vi "Handle Value Change.vi"(5 "VolatusAPI":refnum<class "VolatusAPI.lvclass">, 7 "CtlRef":refnum<vi>, 8 "error in (no error)":errorcluster, 9 "NewVal":variant, 10 "OldVal":variant, 11 "BooleanControl in":refnum<class "BooleanControl.lvclass">) -> (0 "error out":errorcluster, 3 "BooleanControl out":refnum<class "BooleanControl.lvclass">)   [LabVIEW 2020, in "VolatusGUIElements.lvlib" / "BooleanControl.lvclass"]
uses:
  BooleanControl.lvclass
  BooleanControl.lvclass/BooleanControl.ctl
  messages/CmdDigital/Data.ctl
  messages/CmdDigital/CmdDigital.lvlib
  messages/CmdDigital/Class/Msg.lvclass
  Volatus/VolatusAPI/VolatusAPI.lvclass
  VolatusGUI/GUI Element/GUI Element.lvclass
  C:/dev/lv20CE/relink/lv-volatus/messages/CmdDigital/Class/Msg.lvclass
  C:/dev/lv20CE/relink/lv-protoc/LV-Proto/Message/Message.lvclass
  C:/dev/lv20CE/relink/lv-volatus/VolatusGUI/GUI Element/GUI Element.lvclass
  C:/dev/lv20CE/relink/lv-volatus/VolatusGUIElements/BooleanControl/BooleanControl.lvclass
  C:/dev/lv20CE/relink/lv-volatus/VolatusGUI/OnValueChangeHandler/OnValueChangeHandler.lvclass
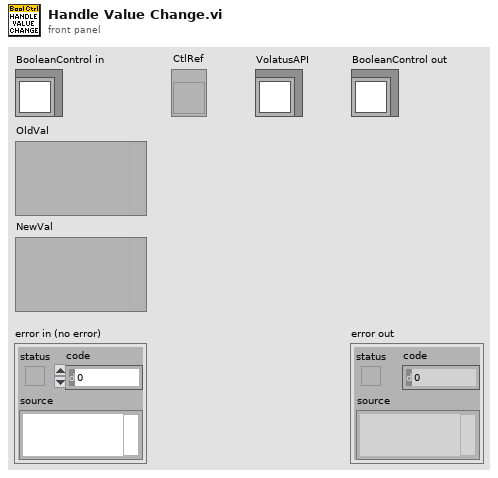
[diagram p1: front panel]
types:
  T1 = typedef "CmdDigital.lvlib/Data.ctl" = cluster{"channel":string, "value":bool}
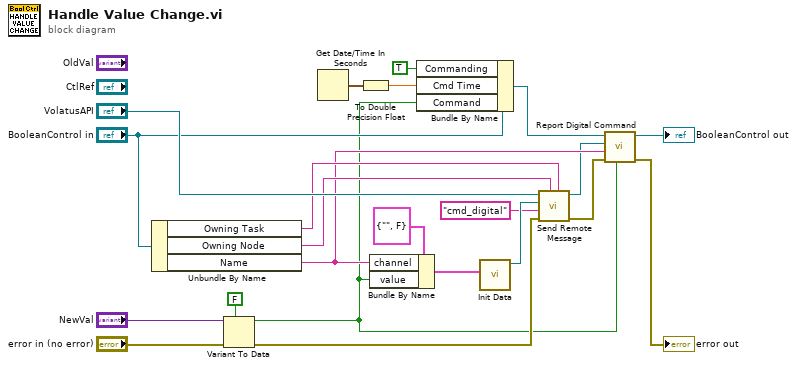
[diagram p0: block diagram]
diagram:
  n1 = Unbundle By Name("BooleanControl in") -> ("Owning Task"=w14:string, "Owning Node"=w13:string, "Name"=w9:string)
  n2 = Variant To Data(error in="error in (no error)", type=FALSE, Variant="NewVal") -> (data=w1:bool, error out=w12:errorcluster)
  n3 = Get Date/Time In Seconds() -> (seconds since 1Jan1904=w4:timestamp)
  n4 = To Double Precision Float(number=w4) -> (double precision float=w3:dbl)
  n5 = Bundle By Name(cluster=T1 {"channel"="", "value"=FALSE} ("Data"), "channel"=w9, "value"=w1) -> (w18:T1)
  n6 = Bundle By Name(cluster="BooleanControl in", "Commanding"=TRUE, "Cmd Time"=w3, "Command"=w1) -> (w5:refnum<class "BooleanControl.lvclass">)
  n7 = call "Init Data.vi"("Data"=w18) -> ("Msg out"=w17:refnum<class "Msg.lvclass">)  [unwired: 10 in]
  n8 = call "Send Remote Message.vi"("Target Task (None)"=w14, "Target Name"=w13, "error in (no error)"=w12, "Message Type"="cmd_digital", "Message"=w17, "VolatusAPI in"="VolatusAPI") -> ("error out"=w8:errorcluster, "VolatusAPI out"=w7:refnum<class "VolatusAPI.lvclass">)  [unwired: 4 in]
  n9 = call "Report Digital Command.vi"("Value"=w1, "error in (no error)"=w8, "Name"=w9, "VolatusAPI in"=w7, "GUI Element in"=w5) -> ("error out"=→"error out":errorcluster, "GUI Element out"=→"BooleanControl out":refnum<class "BooleanControl.lvclass">)  [unwired: 5 in]
